vi "Pad.vi"(9 "size(s)":i32, 10 "block in":u8[](array[numeric]) format="%02x", 11 "Hash Function in":refnum<class "NI_SHA-3.lvclass">) -> (2 "padded input block":u8[](array[numeric]) format="%02x", 3 "Hash Function out":refnum<class "NI_SHA-3.lvclass">)   [LabVIEW 2020, in "NI_SHA-3.lvclass"]
doc: "Prepare a partial input block for input to the hash function."
uses:
  <vilib>/security/Message Digest/SHA-3/NI_SHA-3.lvclass
  <vilib>/security/Message Digest/SHA-3/NI_SHA-3.lvclass/NI_SHA-3.ctl
  0d08caf3-64fe-4c26-8ba2-4be73613850b.vi
  <vilib>/security/Message Digest/SHA-3/Get Block Size.vi
  <vilib>/security/Message Digest/SHA-3/subVIs/Get First Pad Byte.vi
  <vilib>/security/Message Digest/SHA-3/Get Block Size.vi/eb1e6525-3e01-40a8-a5c2-e849aaf68d04.vi
  <vilib>/security/Message Digest/SHA-3/Get Block Size.vi/eb1e6525-3e01-40a8-a5c2-e849aaf68d04.vi/00efce51-7697-47ef-971b-245e50795e7f.vi
  <vilib>/security/Message Digest/SHA-3/subVIs/Get Capacity.vi
  <vilib>/security/Message Digest/SHA-3/subVIs/Get Word Type.vi
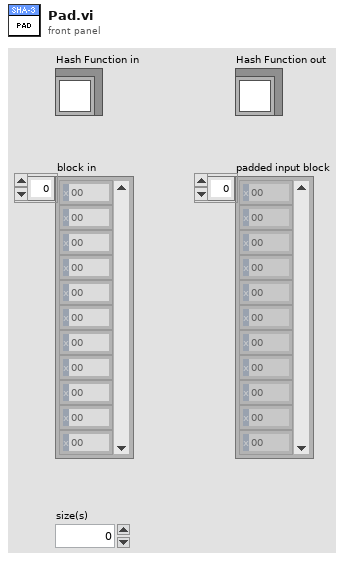
[diagram p1: front panel]
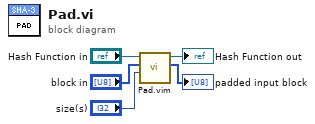
[diagram p0: block diagram]
diagram:
  n1 = call "Pad.vim"("size(s)"="size(s)", "block in"="block in", "Hash Function in"="Hash Function in") -> ("padded input block"=→"padded input block":u8[], "Hash Function out"=→"Hash Function out":refnum<class "NI_SHA-3.lvclass">)  [unwired: 7 in]
